vi "Number of Address Map Elements.vi"(2 "WaveformAddressSpace":refnum<class "WaveformAddressSpace.lvclass">) -> (6 "number of elements":u8)   [LabVIEW 2015, in "WaveformAddressSpace.lvclass"]
uses:
  WaveformAddressSpace.lvclass
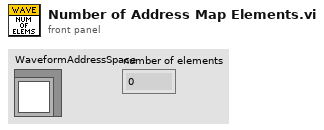
[diagram p1: front panel]
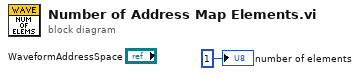
[diagram p0: block diagram]
diagram:
  "number of elements" <- u8 1 ("number of elements")
